vi "parse-modules.vi"(1 "reading":cluster{"address":u16, "value":u16}[](array[cluster])) -> (0 "modules":T1)   [LabVIEW 2021]
uses:
  General Purpose/BMS.ctl
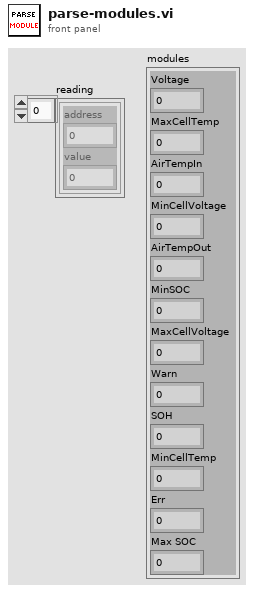
[diagram p1: front panel]
types:
  T1 = cluster{"Voltage":dbl, "MaxCellTemp":dbl, "AirTempIn":dbl, "MinCellVoltage":u16, "AirTempOut":dbl, "MinSOC":u16, "MaxCellVoltage":u16, "Warn":u16, "SOH":u16, "MinCellTemp":dbl, "Err":u16, "Max SOC":u16}
  T2 = typedef "BMS.ctl" = cluster{"rack":cluster{"EoCVoltage":dbl, "MaxChargeCurrent":dbl, "EoDVoltage":dbl, "MaxDischargePower":dbl, "Voltage":dbl, "Current":dbl, "NrOfSRB":u16, "AvgCurrent":dbl, "MaxSOC":u16, "MinSOC":u16, "MaxCellVolt":dbl, "MinCellTemp":dbl, "SOH":u16, "MaxCellTemp":dbl, "AvgCellTemp":dbl, "MinCellVolt":dbl, "MinModVoltage":dbl, "MaxModVoltage":dbl, "Err1":u16, "Warn":u16, "MaxChargePower":dbl, "MaxDischargeCurrent":dbl, "State":string, "ContactorState":string, "OperatingState":string, "Err2":u16}[], "modules":cluster{"Voltage":dbl, "MaxCellTemp":dbl, "AirTempIn":dbl, "MinCellVoltage":u16, "AirTempOut":dbl, "MinSOC":u16, "MaxCellVoltage":u16, "Warn":u16, "SOH":u16, "MinCellTemp":dbl, "Err":u16, "Max SOC":u16}[]}
  T3 = cluster{"Voltage":dbl, "MaxCellTemp":dbl, "AirTempIn":dbl, "MinCellVoltage":u16, "AirTempOut":dbl, "MinSOC":u16, "MaxCellVoltage":u16, "Warn":u16, "SOH":u16, "MinCellTemp":dbl, "Err":u16, "Max SOC":u16}[]
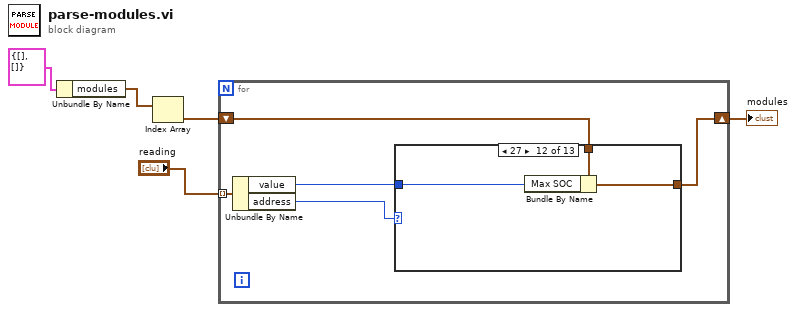
[diagram p0: block diagram]
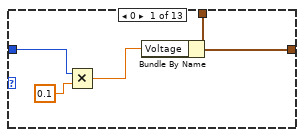
[diagram p2: hidden frame]
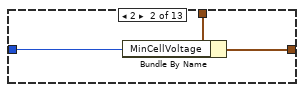
[diagram p3: hidden frame]
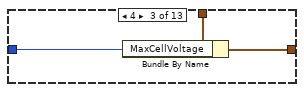
[diagram p4: hidden frame]
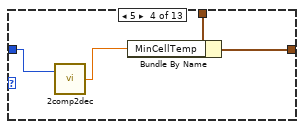
[diagram p5: hidden frame]
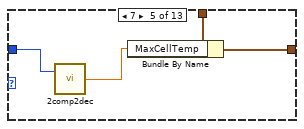
[diagram p6: hidden frame]
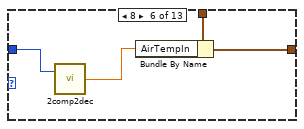
[diagram p7: hidden frame]
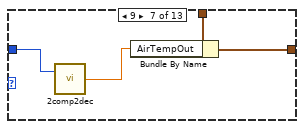
[diagram p8: hidden frame]
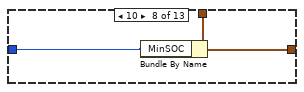
[diagram p9: hidden frame]
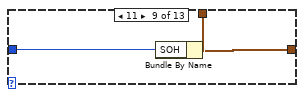
[diagram p10: hidden frame]
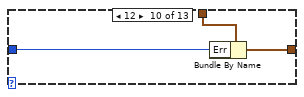
[diagram p11: hidden frame]
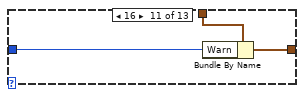
[diagram p12: hidden frame]
diagram:
  n1 = Unbundle By Name(T2 {"rack"=[], "modules"=[]} ("BMS")) -> ("modules"=w2:T3)
  n2 = Index Array(array=w2) -> (element=w3:T1)  [unwired: 1 in]
  n3 = for {
    tunnel: "reading" -> [w10] mode=indexing
    shift-right: [w6] -> w1
    shift-left: w3 -> [w7]
    n4 = Unbundle By Name(w10) -> ("value"=w8:u16, "address"=w9:u16)
    n5 = case shown="27" w9 {
      tunnel: w8 -> [w13 w16 w19 w23 w27 w31 w35 w38 w41 w44 w47 w50 _]
      tunnel: w7 -> [w15 w18 w21 w25 w29 w33 w37 w40 w43 w46 w49 w52 w53]
      tunnel: [w14 w17 w20 w24 w28 w32 w36 w39 w42 w45 w48 w51 w53] -> w6
      frame 0 {
        n6 = Multiply(x=w13, y=0.1) -> (x*y=w12:dbl)
        n7 = Bundle By Name(cluster=w15, "Voltage"=w12) -> (w14:T1)
      }
      frame 2 {
        n8 = Bundle By Name(cluster=w18, "MinCellVoltage"=w16) -> (w17:T1)
      }
      frame 4 {
        n9 = Bundle By Name(cluster=w21, "MaxCellVoltage"=w19) -> (w20:T1)
      }
      frame 5 {
        n10 = call "2comp2dec.vi"("two' complement"=w23) -> ("decimal"=w22:dbl)  [unwired: 2 in]
        n11 = Bundle By Name(cluster=w25, "MinCellTemp"=w22) -> (w24:T1)
      }
      frame 7 {
        n12 = call "2comp2dec.vi"("two' complement"=w27) -> ("decimal"=w26:dbl)  [unwired: 2 in]
        n13 = Bundle By Name(cluster=w29, "MaxCellTemp"=w26) -> (w28:T1)
      }
      frame 8 {
        n14 = call "2comp2dec.vi"("two' complement"=w31) -> ("decimal"=w30:dbl)  [unwired: 2 in]
        n15 = Bundle By Name(cluster=w33, "AirTempIn"=w30) -> (w32:T1)
      }
      frame 9 {
        n16 = call "2comp2dec.vi"("two' complement"=w35) -> ("decimal"=w34:dbl)  [unwired: 2 in]
        n17 = Bundle By Name(cluster=w37, "AirTempOut"=w34) -> (w36:T1)
      }
      frame 10 {
        n18 = Bundle By Name(cluster=w40, "MinSOC"=w38) -> (w39:T1)
      }
      frame 11 {
        n19 = Bundle By Name(cluster=w43, "SOH"=w41) -> (w42:T1)
      }
      frame 12 {
        n20 = Bundle By Name(cluster=w46, "Err"=w44) -> (w45:T1)
      }
      frame 16 {
        n21 = Bundle By Name(cluster=w49, "Warn"=w47) -> (w48:T1)
      }
      frame 27 {
        n22 = Bundle By Name(cluster=w52, "Max SOC"=w50) -> (w51:T1)
      }
      frame Default {
      }
    }
  }
  "modules" <- w1
